vi "Watchdog.vi"(0 "COM Port Select":refnum<visa-resource-name>, 5 "Enable-In":bool=TRUE, 11 "error in (no error)":errorcluster) -> (4 "VISA resource name out":refnum<visa-resource-name>, 6 "WatchDog Status":bool=TRUE, 15 "error out":errorcluster)   [LabVIEW 2020]
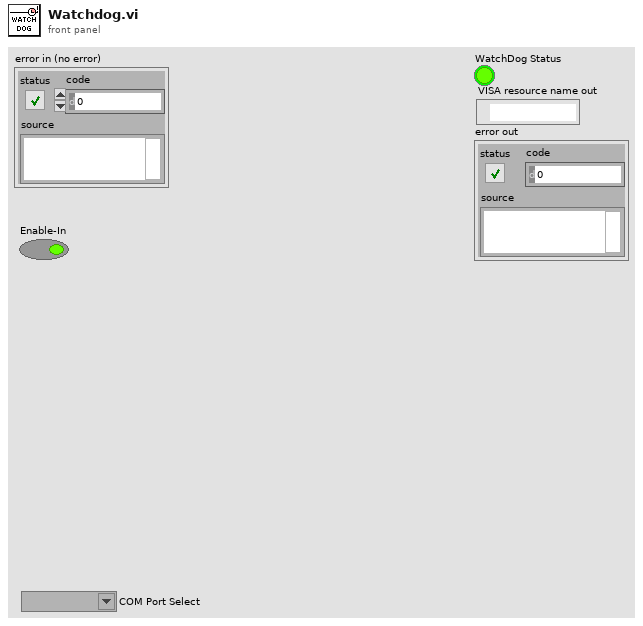
[diagram p1: front panel]
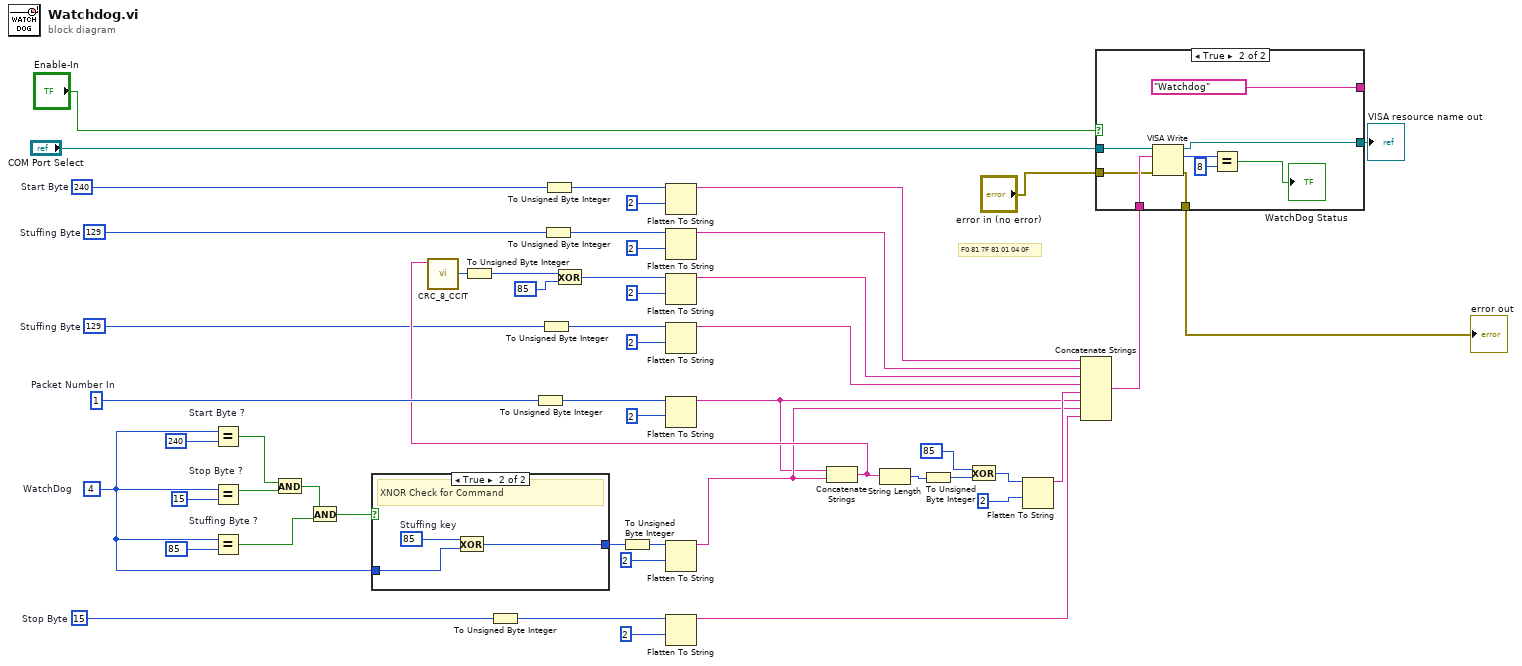
[diagram p0: block diagram]
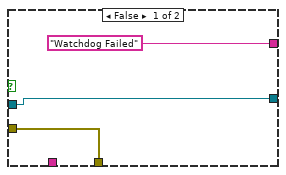
[diagram p2: hidden frame]
diagram:
  w17 = 15  # Stop Byte
  w20 = 129  # Stuffing Byte
  w21 = 129  # Stuffing Byte
  w19 = 240  # Start Byte
  w35 = 4  # WatchDog
  w52 = u8 1  # Packet Number In
  # "F0 81 7F 81 01 04 0F"
  n1 = Equal? "Start Byte ?"(x=w35, y=240 ("IntAck")) -> (x = y?=w8:bool)
  n2 = Equal? "Stop Byte ?"(x=w35, y=15 ("IntAck")) -> (x = y?=w9:bool)
  n3 = Equal? "Stuffing Byte ?"(x=w35, y=85 ("IntAck")) -> (x = y?=w11:bool)
  n4 = And(x=w8, y=w9) -> (x .and. y?=w10:bool)
  n5 = And(x=w10, y=w11) -> (x .and. y?=w12:bool)
  n6 = case shown="True" w12 {
    tunnel: w35 -> [w53 w56]
    tunnel: [w53 w54] -> w36
    frame False {
    }
    frame True {
      w55 = 85  # Stuffing key
      # "XNOR Check for Command"
      n7 = Exclusive Or(1:w56, 2:w55) -> (0:w54:i32)
    }
  }
  n8 = To Unsigned Byte Integer(number=w17) -> (unsigned 8bit integer=w18:u8)
  n9 = To Unsigned Byte Integer(number=w52) -> (unsigned 8bit integer=w43:u8)
  n10 = To Unsigned Byte Integer(number=w21) -> (unsigned 8bit integer=w24:u8)
  n11 = To Unsigned Byte Integer(number=w20) -> (unsigned 8bit integer=w23:u8)
  n12 = To Unsigned Byte Integer(number=w19) -> (unsigned 8bit integer=w22:u8)
  n13 = To Unsigned Byte Integer(number=w36) -> (unsigned 8bit integer=w42:u8)
  n14 = Flatten To String(anything=w22, byte order (0:big-endian, network order)=2) -> (data string=w13:string)  [unwired: 2 in, 2 out]
  n15 = Flatten To String(anything=w23, byte order (0:big-endian, network order)=2) -> (data string=w14:string)  [unwired: 2 in, 2 out]
  n16 = Flatten To String(anything=w24, byte order (0:big-endian, network order)=2) -> (data string=w16:string)  [unwired: 2 in, 2 out]
  n17 = Flatten To String(anything=w43, byte order (0:big-endian, network order)=2) -> (data string=w37:string)  [unwired: 2 in, 2 out]
  n18 = Flatten To String(anything=w42, byte order (0:big-endian, network order)=2) -> (data string=w38:string)  [unwired: 2 in, 2 out]
  n19 = Flatten To String(anything=w18, byte order (0:big-endian, network order)=2) -> (data string=w6:string)  [unwired: 2 in, 2 out]
  n20 = Concatenate Strings(w37, w38) -> (w45:string)
  n21 = call "CRC_8_CCIT.vi"("Data String"=w45) -> ("Numeric"=w44:u8)  [unwired: 10 in]
  n22 = To Unsigned Byte Integer(number=w44) -> (unsigned 8bit integer=w47:u8)
  n23 = Exclusive Or(1:u8 85, 2:w47) -> (0:w46:u8)
  n24 = Flatten To String(anything=w46, byte order (0:big-endian, network order)=2) -> (data string=w15:string)  [unwired: 2 in, 2 out]
  n25 = String Length(string=w45) -> (length=w40:i32)
  n26 = To Unsigned Byte Integer(number=w40) -> (unsigned 8bit integer=w50:u8)
  n27 = Exclusive Or(1:w50, 2:u8 85) -> (0:w49:u8)
  n28 = Flatten To String(anything=w49, byte order (0:big-endian, network order)=2) -> (data string=w41:string)  [unwired: 2 in, 2 out]
  n29 = Concatenate Strings(w13, w14, w15, w16, w41, w37, w38, w6) -> (w7:string)
  n30 = case shown="True" "Enable-In" {
    tunnel: w7 -> [_ w64]
    tunnel: "COM Port Select" -> [w58 w66]
    tunnel: ["Watchdog Failed" "Watchdog"] -> _
    tunnel: [w58 w63] -> w3
    tunnel: "error in (no error)" -> [w57 w62]
    tunnel: [w57 w61] -> w1
    frame False {
    }
    frame True {
      n31 = VISA Write(VISA resource name=w66, write buffer=w64, error in (no error)=w62) -> (VISA resource name out=w63:refnum<visa-resource-name>, return count=w68:u32, error out=w61:errorcluster)
      n32 = Equal?(x=w68, y=u32 8) -> (x = y?=→"WatchDog Status":bool)
    }
  }
  "VISA resource name out" <- w3
  "error out" <- w1
